vi "Main Page.vi"(8 "error in (no error)":errorcluster, 11 "Node Ptr":T1 format="%.0x") -> (0 "error out":errorcluster)   [LabVIEW 2017, in "SLSC Switch System Explorer.lvlib"]
uses:
  SLSC Switch System Explorer.lvlib
  <vilib>/NI Veristand/Custom Device API/Custom Device Item Ref.ctl
  Main Page Controls.ctl
  <vilib>/NI Veristand/Custom Device API/Custom Device API.lvlib
  Scripting/SLSC Switch Scripting.lvlib
panel:
  in  "Topology":string(combo)
  out "Resource Name":string
  out "Model Number":string
  in  "SHDocVw.IWebBrowser":refnum<k7>(container)
  in  "Description":string
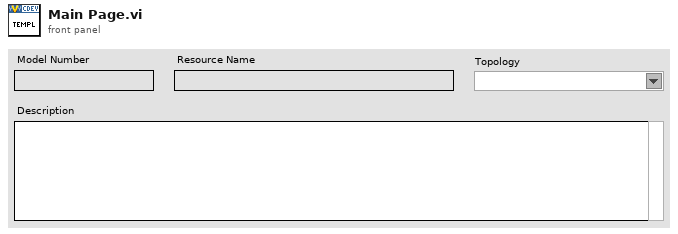
[diagram p1: front panel]
types:
  T1 = typedef "Custom Device API.lvlib/Custom Device Item Ref.ctl" = u64
  T2 = typedef "SLSC Switch System Explorer.lvlib/Main Page Controls.ctl" = cluster{"Description":refnum<vi>, "Model Number":refnum<vi>, "Resource Name":refnum<vi>, "Topology":refnum<vi>}
  T3 = typedef "Custom Device API.lvlib/Custom Device Commands.ctl" = enum16{"Default", "Item renamed", "Shutdown", "Dynamic button pressed"}
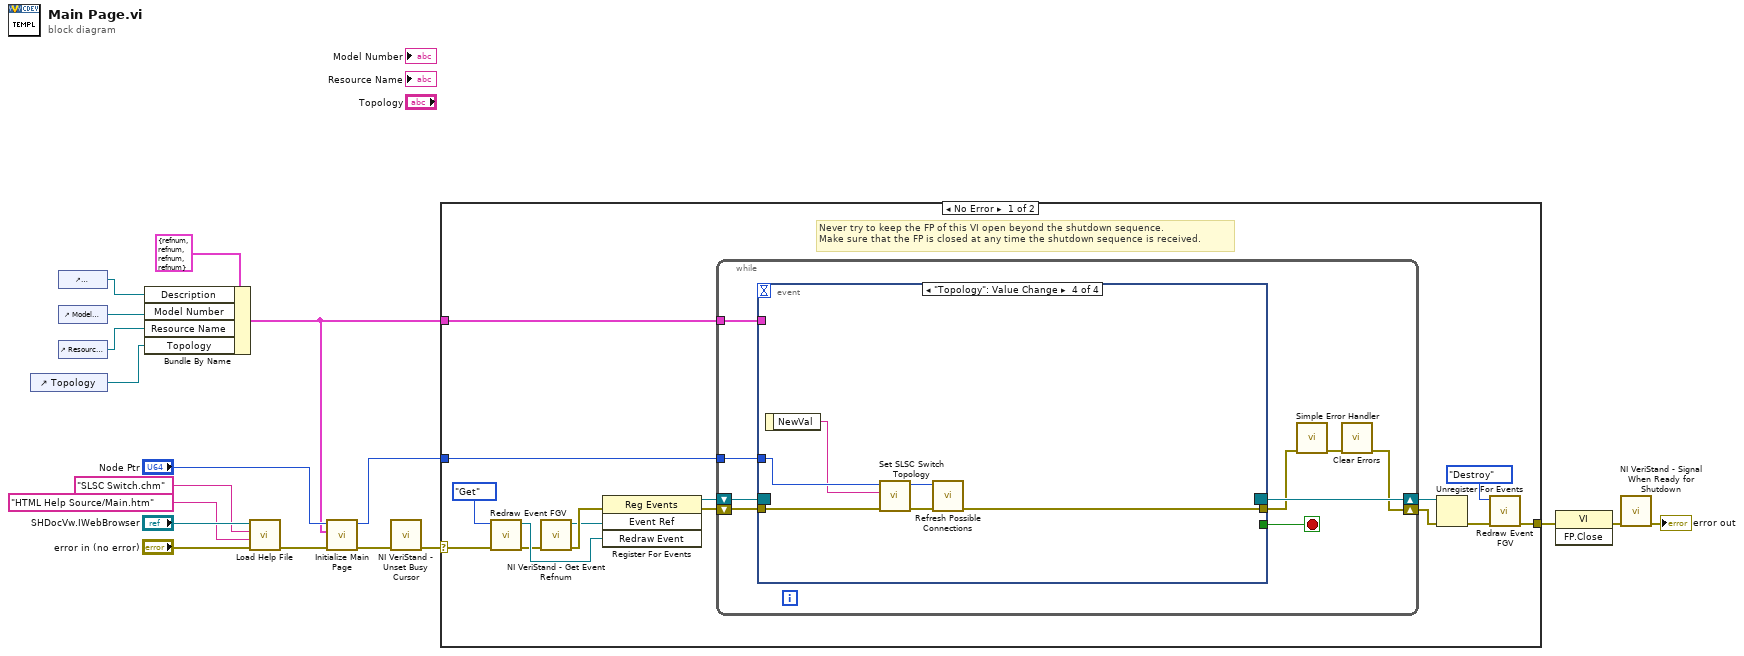
[diagram p0: block diagram]
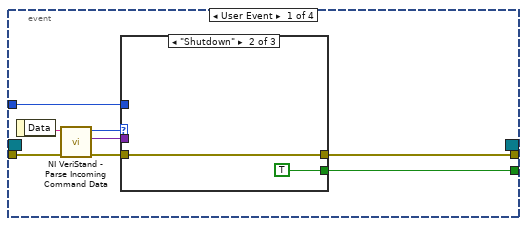
[diagram p2: hidden frame]
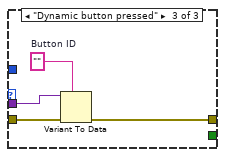
[diagram p4: hidden frame]
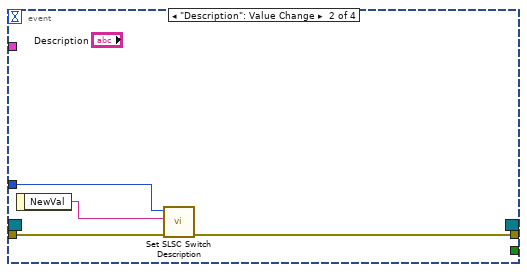
[diagram p5: hidden frame]
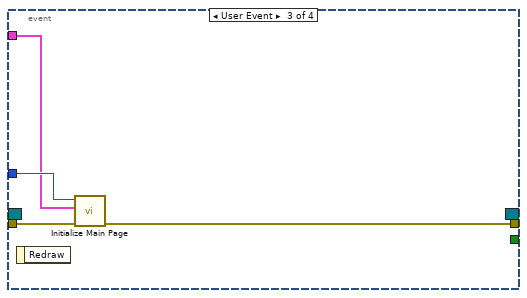
[diagram p6: hidden frame]
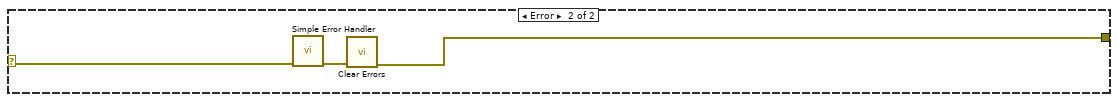
[diagram p7: hidden frame]
diagram:
  n1 = control-ref of="Topology"() -> (w4:refnum<vi>)
  n2 = control-ref of="Description"() -> (w7:refnum<vi>)
  n3 = control-ref of="Model Number"() -> (w3:refnum<vi>)
  n4 = control-ref of="Resource Name"() -> (w2:refnum<vi>)
  n5 = Bundle By Name(cluster=T2 {"Description"=refnum, "Model Number"=refnum, "Resource Name"=refnum, "Topology"=refnum} ("Main Page Controls"), "Description"=w7, "Model Number"=w3, "Resource Name"=w2, "Topology"=w4) -> (w1:T2)
  n6 = call "Load Help File.vi"("error in (no error)"="error in (no error)", "HTML File to Load"="HTML Help Source/Main.htm" ("HTML File"), "Main CHM File"="SLSC Switch.chm" ("CD_CHM_FileName"), "Browser"="SHDocVw.IWebBrowser") -> ("error out"=w5:errorcluster)  [unwired: 7 in]
  n7 = call "Initialize Main Page.vi"("error in (no error)"=w5, "Main Page Controls"=w1, "Item Ref in"="Node Ptr") -> ("error out"=w14:errorcluster, "Item Ref out"=w11:T1)  [unwired: 7 in]
  n8 = call <vilib>:"NI VeriStand - Unset Busy Cursor.vi"("error in (no error)"=w14) -> ("error out"=w13:errorcluster)  [unwired: 10 out]
  n9 = case shown="No Error" w13 {
    selector: w13 -> [w21 w74]
    tunnel: [w23 w72] -> w18
    tunnel: w11 -> [w27 _]
    tunnel: w1 -> [w25 _]
    frame No Error {
      # "Never try to keep the FP of this VI open beyond the shutdown sequence.\nMake sure that the FP is closed at any time the shutdown sequence is received."
      n10 = call "Redraw Event FGV.vi"("error in (no error)"=w21, "Action (Get)"=enum16{"Get", "Destroy"}."Get") -> ("error out"=w20:errorcluster, "Redraw Event"=w26:refnum<user-event>)  [unwired: 8 in]
      n11 = call <vilib>:"NI VeriStand - Get Event Refnum.vi"("error in (no error)"=w20) -> ("error out"=w33:errorcluster, "Event Ref"=w30:refnum<user-event>)  [unwired: 9 out]
      n12 = register-events(error in=w33, w30, w26) -> (reference out=w28:refnum<event-registration>, error out=w29:errorcluster)  [unwired: 1 in]
      n13 = while {
        tunnel: w27 -> [w38]
        shift-right: [w35] -> w31
        shift-left: w29 -> [w41]
        shift-right: [w42] -> w32
        shift-left: w28 -> [w40]
        tunnel: w25 -> [w34]
        stop <- w39 stop-if-true
        n14 = event shown="[3] \"Topology\": Value Change" {
          selector: w40 -> [_ _ _ _]
          dyn-events: [_ _ _ _] -> w42
          timeout: _ -> [_ _ _ _]
          tunnel: w41 -> [w50 w60 w63 w71]
          tunnel: [w46 _ _ _] -> w39
          tunnel: [w45 w59 w62 w68] -> w37
          tunnel: w38 -> [w44 w61 w65 w70]
          tunnel: w34 -> [_ _ w64 _]
          event User Event {
            n15 = event-data() -> ("Data"=w49:string)  [unwired: 1 out]
            n16 = call <vilib>:"NI VeriStand - Parse Incoming Command Data.vi"("error in (no error)"=w50, "Incoming data"=w49) -> ("error out"=w48:errorcluster, "Outgoing data"=w43:variant, "Action"=w47:T3)  [unwired: 7 out]
            n17 = case shown="\"Shutdown\"" w47 {
              tunnel: w48 -> [w51 w52 w57]
              tunnel: [_ TRUE _] -> w46
              tunnel: [w51 w52 w54] -> w45
              tunnel: w44 -> [_ _ _]
              tunnel: w43 -> [_ _ w56]
              frame "Default", Default {
              }
              frame "Shutdown" {
              }
              frame "Dynamic button pressed" {
                w55 = ""  # Button ID
                n18 = Variant To Data(error in=w57, type=w55, Variant=w56) -> (error out=w54:errorcluster)  [unwired: 1 out]
              }
            }
          }
          event "Description": Value Change {
            n19 = event-data() -> ("NewVal"=w58:string)  [unwired: 1 out]
            n20 = call "Set SLSC Switch Description.vi"("error in (no error)"=w60, "Description"=w58, "SLSC Switch Custom Device Ref in"=w61) -> ("error out"=w59:errorcluster)  [unwired: 7 in, 1 out]
          }
          event User Event {
            n21 = event-data() -> ()  [unwired: 2 out]
            n22 = call "Initialize Main Page.vi"("error in (no error)"=w63, "Main Page Controls"=w64, "Item Ref in"=w65) -> ("error out"=w62:errorcluster)  [unwired: 7 in, 1 out]
          }
          event "Topology": Value Change {
            n23 = event-data() -> ("NewVal"=w69:string)  [unwired: 1 out]
            n24 = call "Set SLSC Switch Topology.vi"("error in (no error)"=w71, "Topology"=w69, "SLSC Switch Custom Device Ref in"=w70) -> ("error out"=w66:errorcluster, "SLSC Switch Custom Device Ref out"=w67:T1)  [unwired: 7 in]
            n25 = call "Refresh Possible Connections.vi"("error in (no error)"=w66, "SLSC Switch Custom Device Ref in"=w67) -> ("error out"=w68:errorcluster)  [unwired: 8 in, 1 out]
          }
        }
        n26 = call <vilib>:"Simple Error Handler.vi"("error in (no error)"=w37) -> ("error out"=w36:errorcluster)  [unwired: 1 in, 7 out]
        n27 = call <vilib>:"Clear Errors.vi"("error in (no error)"=w36) -> ("error out"=w35:errorcluster)  [unwired: 1 in, 5 out]
      }
      n28 = Unregister For Events(event registration refnum=w32, error in=w31) -> (error out=w24:errorcluster)
      n29 = call "Redraw Event FGV.vi"("error in (no error)"=w24, "Action (Get)"=enum16{"Get", "Destroy"}."Destroy") -> ("error out"=w23:errorcluster)  [unwired: 8 in, 1 out]
    }
    frame Error {
      n30 = call <vilib>:"Simple Error Handler.vi"("error in (no error)"=w74) -> ("error out"=w73:errorcluster)  [unwired: 1 in, 7 out]
      n31 = call <vilib>:"Clear Errors.vi"("error in (no error)"=w73) -> ("error out"=w72:errorcluster)  [unwired: 1 in, 5 out]
    }
  }
  n32 = invoke class="VI" method="FP.Close"(error in=w18) -> (error out=w17:errorcluster)  [unwired: 2 in, 2 out]
  n33 = call <vilib>:"NI VeriStand - Signal When Ready for Shutdown.vi"("error in (no error)"=w17) -> ("error out"=→"error out":errorcluster)  [unwired: 10 out]
